vi "Get Properties.vi"(8 "error in (no error)":errorcluster, 11 "TTLControl in":refnum<class "TTLController.lvclass">) -> (0 "error out":errorcluster, 2 "Properties":string[](array[string]), 3 "TTLControl out":refnum<class "TTLController.lvclass">)   [LabVIEW 2020, in "TTLController.lvclass"]
uses:
  TTLController.lvclass
  TTLController.lvclass/TTLController.ctl
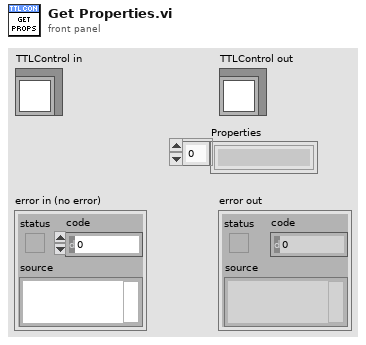
[diagram p1: front panel]
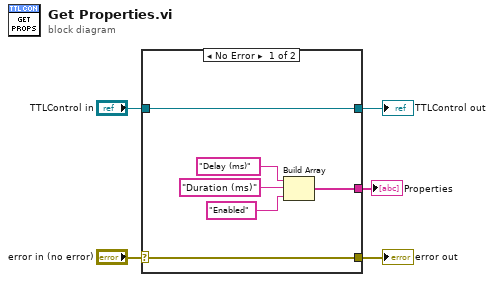
[diagram p0: block diagram]
diagram:
  n1 = case shown="No Error" "error in (no error)" {
    selector: "error in (no error)" -> [w10 w13]
    tunnel: [w10 w13] -> w4
    tunnel: [w11 w12] -> w2
    tunnel: "TTLControl in" -> [w11 w12]
    tunnel: [w6 _] -> w1
    frame No Error {
      n2 = Build Array("Delay (ms)", "Duration (ms)", "Enabled" ("element")) -> (w6:string[])
    }
    frame Error {
    }
  }
  "error out" <- w4
  "TTLControl out" <- w2
  "Properties" <- w1
